vi "VisualInspectionAHU.vi"(8 "error in (no error)":errorcluster, 11 "TableRef":refnum<vi>) -> (0 "error out":errorcluster, 2 "VisualInspectionResult":bool)   [LabVIEW 2017]
panel:
  in  "14.3":dbl
  in  "11":dbl
  in  "15.1":dbl
  in  "14.2":dbl
  in  "14.1":dbl
  in  "13.2":dbl
  in  "13.1":dbl
  in  "12.1":dbl
  in  "10.4":dbl
  in  "10.3":dbl
  in  "10.2":dbl
  in  "10.1":dbl
  in  "9.1":dbl
  in  "16":bool
  in  "8.2":bool
  in  "8.1":bool
  in  "Cancel Button":bool
  in  "OK Button":bool
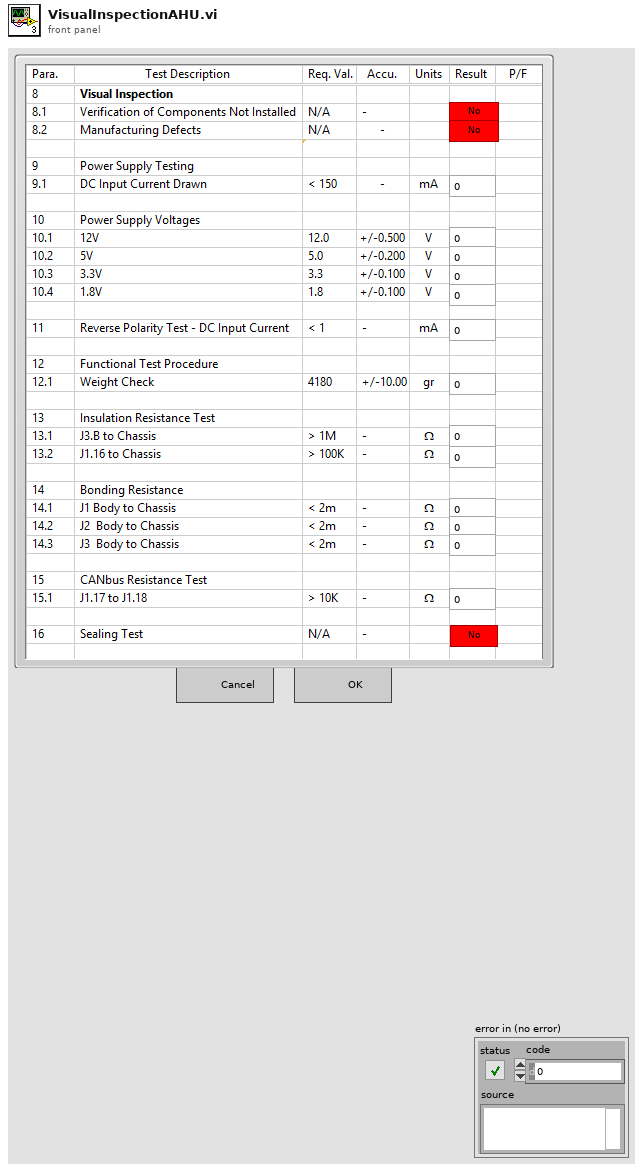
[diagram p1: front panel]
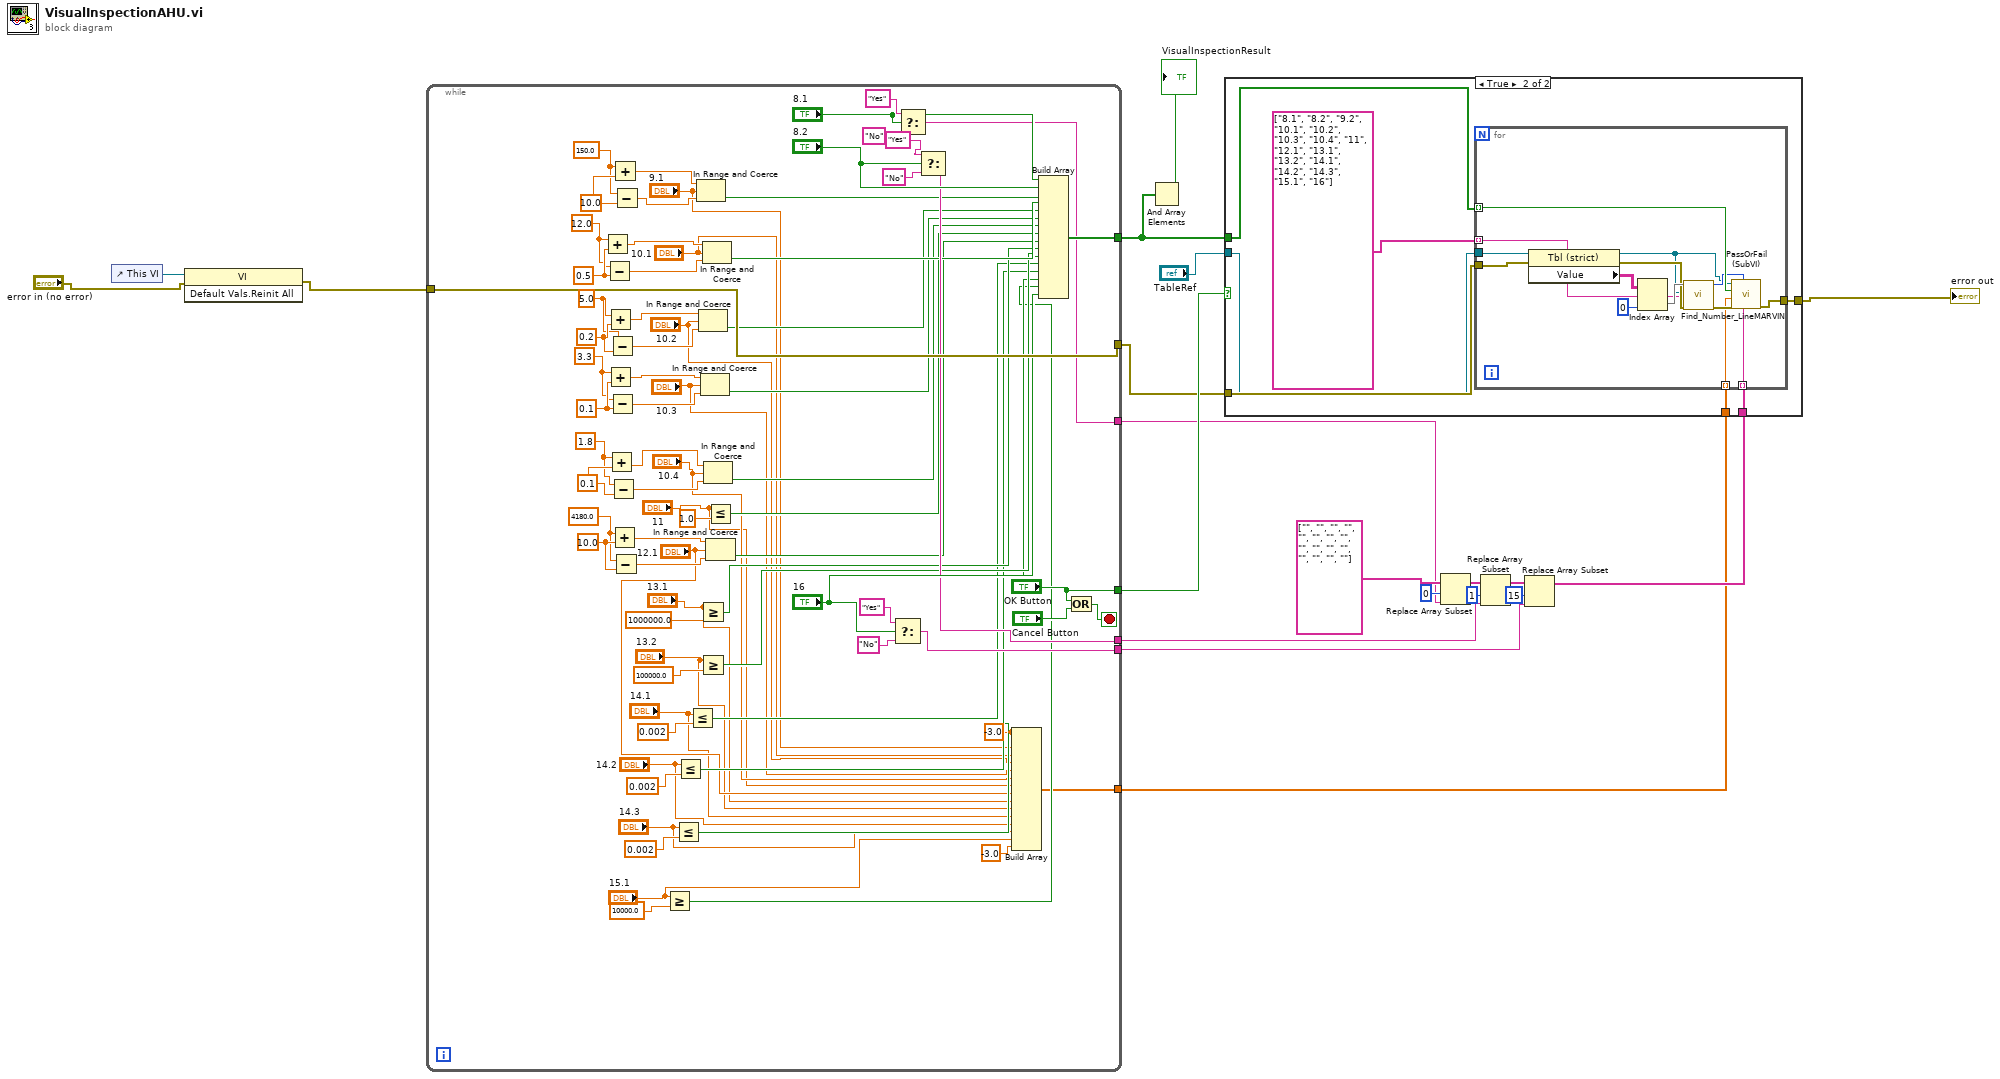
[diagram p0: block diagram]
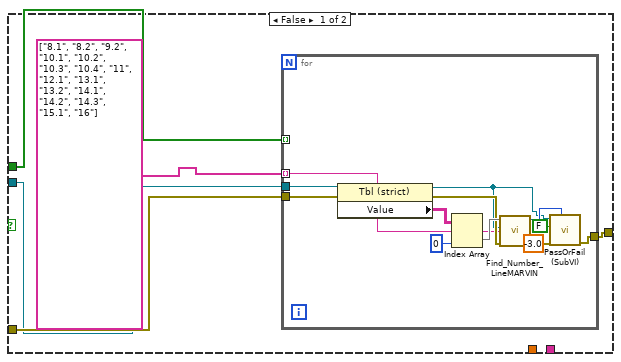
[diagram p2: hidden frame]
diagram:
  n1 = control-ref of="This VI"() -> (w16:refnum<vi>)
  n2 = invoke class="VI" method="Default Vals.Reinit All"(reference=w16, error in="error in (no error)") -> (error out=w20:errorcluster)  [unwired: 1 in, 2 out]
  n3 = while {
    tunnel: w20 -> [w93]
    tunnel: [w95] -> w13
    tunnel: ["OK Button"] -> w19
    tunnel: [w93] -> w18
    tunnel: [w53] -> w5
    tunnel: [w52] -> w4
    tunnel: [w51] -> w3
    tunnel: [w21] -> w1
    stop <- w96 stop-if-true
    w36 = -3.0 ("element")
    w72 = 0.5 ("y")
    w74 = 0.2 ("y")
    w76 = 0.1 ("y")
    w78 = 0.1 ("y")
    w80 = 10.0 ("y")
    w70 = 10.0 ("y")
    w79 = 4180.0 ("y")
    w77 = 1.8 ("y")
    w75 = 3.3 ("y")
    w73 = 5.0 ("y")
    w71 = 12.0 ("y")
    w69 = 150.0 ("y")
    n4 = Add(x=w71, y=w72) -> (x+y=w83:dbl)
    n5 = Subtract(x=w71, y=w72) -> (x-y=w84:dbl)
    n6 = Add(x=w73, y=w74) -> (x+y=w85:dbl)
    n7 = Add(x=w75, y=w76) -> (x+y=w87:dbl)
    n8 = Add(x=w77, y=w78) -> (x+y=w89:dbl)
    n9 = Subtract(x=w73, y=w74) -> (x-y=w86:dbl)
    n10 = Subtract(x=w75, y=w76) -> (x-y=w88:dbl)
    n11 = Subtract(x=w77, y=w78) -> (x-y=w90:dbl)
    n12 = Add(x=w79, y=w80) -> (x+y=w91:dbl)
    n13 = Add(x=w69, y=w70) -> (x+y=w81:dbl)
    n14 = Subtract(x=w79, y=w80) -> (x-y=w92:dbl)
    n15 = Subtract(x=w69, y=w70) -> (x-y=w82:dbl)
    n16 = Greater Or Equal?(x="15.1", y=10000.0) -> (x >= y?=w37:bool)
    n17 = Less Or Equal?(x="14.3", y=0.002) -> (x <= y?=w38:bool)
    n18 = Less Or Equal?(x="14.2", y=0.002) -> (x <= y?=w39:bool)
    n19 = Less Or Equal?(x="14.1", y=0.002) -> (x <= y?=w40:bool)
    n20 = In Range and Coerce(upper limit=w81, x="9.1", lower limit=w82) -> (In Range?=w49:bool)  [unwired: 1 out]
    n21 = In Range and Coerce(upper limit=w85, x="10.2", lower limit=w86) -> (In Range?=w47:bool)  [unwired: 1 out]
    n22 = Greater Or Equal?(x="13.1", y=1000000.0) -> (x >= y?=w42:bool)
    n23 = Greater Or Equal?(x="13.2", y=100000.0) -> (x >= y?=w41:bool)
    n24 = In Range and Coerce(upper limit=w87, x="10.3", lower limit=w88) -> (In Range?=w46:bool)  [unwired: 1 out]
    n25 = In Range and Coerce(upper limit=w83, x="10.1", lower limit=w84) -> (In Range?=w48:bool)  [unwired: 1 out]
    n26 = In Range and Coerce(upper limit=w89, x="10.4", lower limit=w90) -> (In Range?=w45:bool)  [unwired: 1 out]
    n27 = Less Or Equal?(x="11", y=1.0) -> (x <= y?=w44:bool)
    n28 = In Range and Coerce(upper limit=w91, x="12.1", lower limit=w92) -> (In Range?=w43:bool)  [unwired: 1 out]
    n29 = Select(t="Yes", s="16", f="No") -> (s? t:f=w51:string)
    n30 = Select(t="Yes", s="8.1", f="No") -> (s? t:f=w53:string)
    n31 = Select(t="Yes", s="8.2", f="No") -> (s? t:f=w52:string)
    n32 = Build Array(w36, w36, "9.1", "10.1", "10.2", "10.3", "10.4", "11", "12.1", "13.1", "13.2", "14.1", "14.2", "14.3", "15.1", -3.0 ("element")) -> (w21:dbl[])
    n33 = Build Array("8.1", "8.2", w49, w48, w47, w46, w45, w44, w43, w42, w41, w40, w39, w38, w37, "16") -> (w95:bool[])
    n34 = Or(x="OK Button", y="Cancel Button") -> (x .or. y?=w96:bool)
  }
  n35 = And Array Elements(Boolean array=w13) -> (logical AND=→"VisualInspectionResult":bool)
  n36 = Replace Array Subset(array=string[] ["", "", "", "", "", "", "", "", "", "", "", "", "", "", "", ""], new element=w5, index=0) -> (w10:string[])
  n37 = Replace Array Subset(array=w10, new element=w4, index=1) -> (w9:string[])
  n38 = Replace Array Subset(array=w9, new element=w3, index=15) -> (w2:string[])
  n39 = case shown="True" w19 {
    tunnel: w13 -> [w102 w122]
    tunnel: w18 -> [w101 w121]
    tunnel: [w100 w120] -> w14
    tunnel: "TableRef" -> [w99 w119]
    tunnel: w2 -> [_ w117]
    tunnel: w1 -> [_ w116]
    frame False {
      n40 = for {
        tunnel: string[] ["8.1", "8.2", "9.2", "10.1", "10.2", "10.3", "10.4", "11", "12.1", "13.1", "13.2", "14.1", "14.2", "14.3", "15.1", "16"] ("Array 3") -> [w111] mode=indexing
        tunnel: w102 -> [_] mode=indexing
        tunnel: w101 -> [w108]
        tunnel: [w107] -> w100
        tunnel: w99 -> [w106]
        n41 = property class="Tbl (strict)"(reference=w106, error in=w108) -> (reference out=w103:refnum<vi>, error out=w112:errorcluster, "Value"=w115:string[][])
        n42 = Index Array(array=w115, index (col)=0 ("disabled index (col)")) -> (element=w113:string[])  [unwired: 1 in]
        n43 = call "Find_Number_LineMARVIN.vi"("Test Paragraph"=w111, "error in"=w112, "TableIn"=w103, "Row Headers[]"=w113) -> ("error out"=w110:errorcluster, "Line number"=w109:i32)  [unwired: 1 in, 2 out]
        n44 = call "PassOrFail (SubVI).vi"("index (row)"=w109, "error in (no error)"=w110, "Data in"=-3.0, "Pass?Fail"=FALSE ("Boolean"), "Table in"=w103) -> ("error out"=w107:errorcluster)  [unwired: 6 in]
      }
    }
    frame True {
      n45 = for {
        tunnel: string[] ["8.1", "8.2", "9.2", "10.1", "10.2", "10.3", "10.4", "11", "12.1", "13.1", "13.2", "14.1", "14.2", "14.3", "15.1", "16"] ("Array 3") -> [w132] mode=indexing
        tunnel: w122 -> [w130] mode=indexing
        tunnel: w121 -> [w128]
        tunnel: [w127] -> w120
        tunnel: w119 -> [w126]
        tunnel: w117 -> [w124] mode=indexing
        tunnel: w116 -> [w123] mode=indexing
        n46 = property class="Tbl (strict)"(reference=w126, error in=w128) -> (reference out=w125:refnum<vi>, error out=w133:errorcluster, "Value"=w136:string[][])
        n47 = Index Array(array=w136, index (col)=0 ("disabled index (col)")) -> (element=w134:string[])  [unwired: 1 in]
        n48 = call "Find_Number_LineMARVIN.vi"("Test Paragraph"=w132, "error in"=w133, "TableIn"=w125, "Row Headers[]"=w134) -> ("error out"=w131:errorcluster, "Line number"=w129:i32)  [unwired: 1 in, 2 out]
        n49 = call "PassOrFail (SubVI).vi"("String Res"=w124, "index (row)"=w129, "error in (no error)"=w131, "Data in"=w123, "Pass?Fail"=w130, "Table in"=w125) -> ("error out"=w127:errorcluster)  [unwired: 5 in]
      }
    }
  }
  "error out" <- w14
